vi "fgv_DS1202_config.vi"(7 "cmd":T2, 11 "config":T1={"VISA "="USB0::0x1AB1::0x0517::DS1ZE244412916::INSTR", "Timeout"=10000, "Channel"=0} {"Channel" items=["Channel 1", "Channel 2", "Channel 3", "Channel 4"]}) -> (3 "config 2":T1={"VISA "="USB0::0x1AB1::0x0517::DS1ZE244412916::INSTR", "Timeout"=10000, "Channel"=0} {"Channel" items=["Channel 1", "Channel 2", "Channel 3", "Channel 4"]})   [LabVIEW 2021]
uses:
  ctrl/rw.ctl
  ctrl/DS1202_cfg.ctl
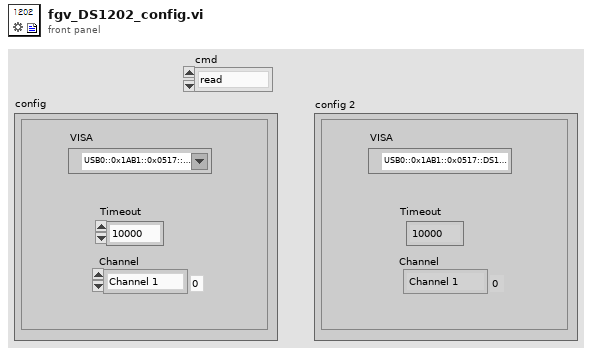
[diagram p1: front panel]
types:
  T1 = typedef "DS1202_cfg.ctl" = cluster{"VISA ":refnum<visa-resource-name>, "Timeout":u32, "Channel":u16}
  T2 = typedef "rw.ctl" = enum16{"read", "write"}
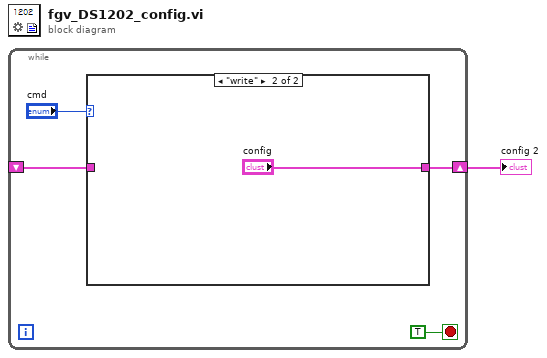
[diagram p0: block diagram]
diagram:
  n1 = while {
    shift-right: [w3] -> w1
    shift-left: _ -> [w2]
    stop <- TRUE stop-if-true
    n2 = case shown="\"write\"" "cmd" {
      tunnel: [w6 "config"] -> w3
      tunnel: w2 -> [w6 _]
      frame "read", Default {
      }
      frame "write" {
      }
    }
  }
  "config 2" <- w1
